vi "Pause.vi"(8 "error in (no error)":errorcluster, 11 "Wait in":refnum<class "Wait.lvclass">) -> (0 "error out":errorcluster, 3 "Wait out":refnum<class "Wait.lvclass">)   [LabVIEW 2019, in "Wait.lvclass"]
uses:
  <vilib>/gpm_packages/@cs/Car-wash/Source/Process Steps/Wait/Wait.lvclass
  <vilib>/ActorFramework/Time-Delayed Send Message/Time-Delay Override Options.ctl
  <vilib>/gpm_packages/@cs/Car-wash/Source/Process Steps/Wait/Wait.lvclass/Wait.ctl
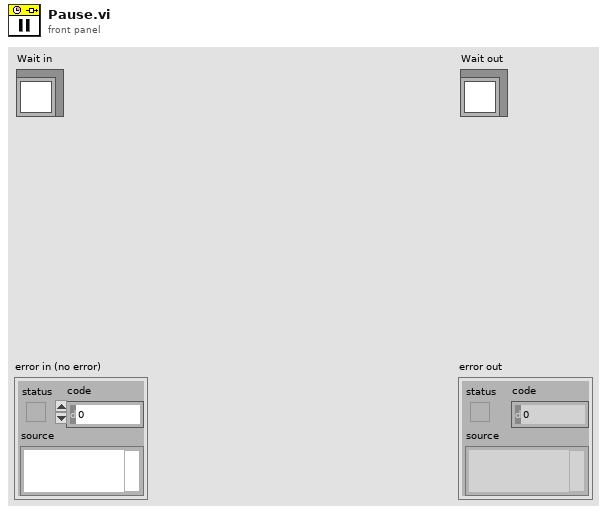
[diagram p1: front panel]
types:
  T1 = typedef "Time-Delay Override Options.ctl" = enum16{"Send next copy now", "Skip next scheduled copy", "Send next copy now and stop all further copies", "Stop all further copies"}
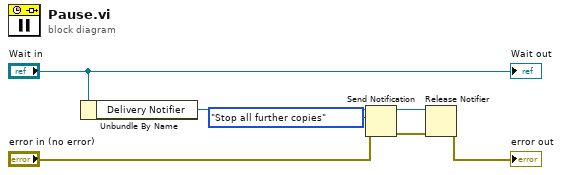
[diagram p0: block diagram]
diagram:
  n1 = Unbundle By Name("Wait in") -> ("Delivery Notifier"=w6:refnum<notifier>)
  n2 = Send Notification(notification=Time-Delay_Override_Options."Stop all further copies", notifier=w6, error in (no error)="error in (no error)") -> (notifier out=w3:refnum<notifier>, error out=w2:errorcluster)
  n3 = Release Notifier(notifier=w3, error in (no error)=w2) -> (error out=→"error out":errorcluster)  [unwired: 1 in, 2 out]
  "Wait out" <- "Wait in"
